vi "Get Position Display Resolution.vi"(4 "error in (no error)":errorcluster, 6 "Axis (1)":i32=1 min=1 max=3, 7 "VISA resource name":refnum<visa-resource-name>) -> (0 "error out":errorcluster, 2 "Display Resolution":i32, 3 "VISA resource name out":refnum<visa-resource-name>)   [LabVIEW 2015, in "Newport ESP301.lvlib"]
doc: "Reads the display resolution of position information.\nIf Display Resolution = 4 the diplay will show values as low as 0.0001 units.\nIf Display Resolution = 7 the diplay will show values in exponential form as 1.000000E+0 units."
uses:
  Newport ESP301.lvlib
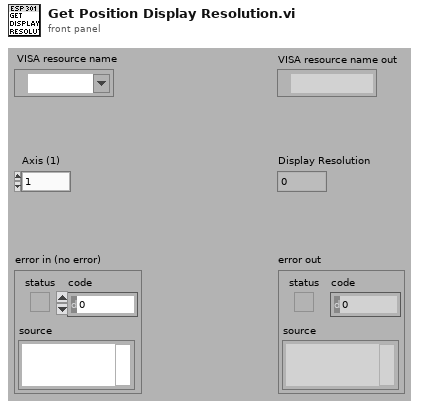
[diagram p1: front panel]
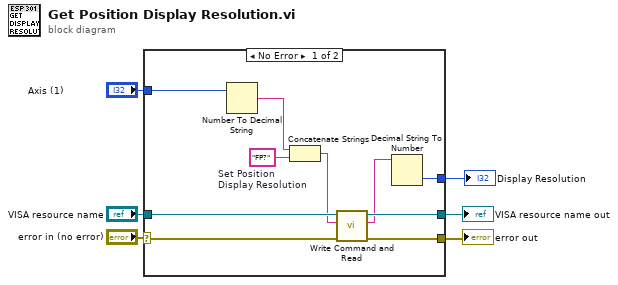
[diagram p0: block diagram]
diagram:
  n1 = case shown="No Error" "error in (no error)" {
    selector: "error in (no error)" -> [w13 w18]
    tunnel: [w15 w18] -> w6
    tunnel: "VISA resource name" -> [w16 w17]
    tunnel: [w14 w17] -> w5
    tunnel: "Axis (1)" -> [w9 _]
    tunnel: [w7 _] -> w1
    frame No Error {
      w12 = "FP?"  # Set Position  Display Resolution
      n2 = Number To Decimal String(number=w9) -> (decimal integer string=w11:string)  [unwired: 1 in]
      n3 = Concatenate Strings(w11, w12) -> (w10:string)
      n4 = call "Write Command and Read.vi"("error in (no error)"=w13, "Command"=w10, "VISA resource name"=w16) -> ("error out"=w15:errorcluster, "Returned string"=w8:string, "VISA resource name out"=w14:refnum<visa-resource-name>)  [unwired: 4 in]
      n5 = Decimal String To Number(string=w8) -> (number=w7:i32)  [unwired: 2 in, 1 out]
    }
    frame Error {
    }
  }
  "error out" <- w6
  "VISA resource name out" <- w5
  "Display Resolution" <- w1
